vi "Ultrasonic.vi"() -> ()   [LabVIEW 2016, in "ENED1100-UCBA-Sensor-Motor-Testing.lvrbt"]
uses:
  ENED1100-UCBA-Sensor-Motor-Testing.lvrbt
  <vilib>/NXT/Block Support/NXT_InputPort.ctl
  <vilib>/NXT/Subs/LVHSConnector.ctl
  <vilib>/NXT/LegoClasses/BrickReference/BrickReference.lvclass
  <vilib>/NXT/Dual Mode Library/Sensors/EV3_Ultrasonic_CM.vi
  <vilib>/NXT/Dual Mode Library/Sound/PlayF.vi
  <vilib>/NXT/Dual Mode Library/Sound/PlayC.vi
panel:
  out "NXT/EV3 4":T1
  in  "NXT/EV3 3":T1
  in  "Port (Port 3) 2":T2=3 items=["Port 1", "Port 2", "Port 3", "Port 4"]
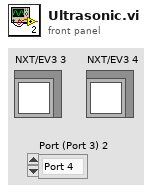
[diagram p1: front panel]
types:
  T1 = typedef "LVHSConnector.ctl" = refnum<class "BrickReference.lvclass">
  T2 = typedef "NXT_InputPort.ctl" = u32
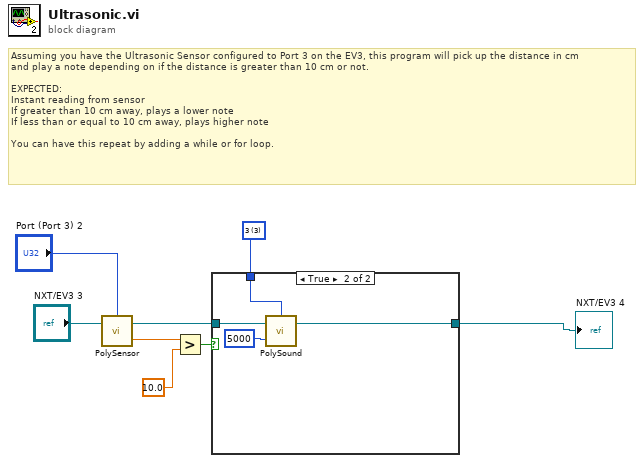
[diagram p0: block diagram]
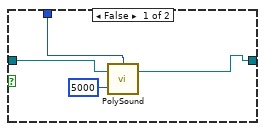
[diagram p2: hidden frame]
diagram:
  w3 = u16 3 items=["3"=3, "4"=4, "5"=5, "6"=6, "7"=7] ("Octave")
  # "Assuming you have the Ultrasonic Sensor configured to Port 3 on the EV3, this program will pick up the distance in cm\nand play a note depending on if the distance is greater than 10 cm or not.\n\nEXPECTED:\nInstant reading from sensor\nIf greater than 10 cm away, plays a lower note\nIf less than or equal to 10 cm away, plays higher note\n\nYou can have this repeat by adding a while or for loop."
  n1 = call-poly <vilib>:"PolySensor.vi"("NXT/EV3"="NXT/EV3 3", "Port (Port 1)"="Port (Port 3) 2") -> ("Centimeters"=w2:sgl, "NXT/EV3"=w5:T1)  [unwired: 1 in]
  n2 = Greater?(x=w2, y=sgl 10.0) -> (0:w6:bool)
  n3 = case shown="True" w6 {
    tunnel: w5 -> [w12 w16]
    tunnel: [w11 w14] -> w4
    tunnel: w3 -> [w10 w13]
    frame False {
      n4 = call-poly <vilib>:"PolySound.vi"("Duration (500 ms)"=u16 5000, "NXT/EV3"=w12, "Octave"=w10) -> ("NXT/EV3"=w11:T1)  [unwired: 1 in]
    }
    frame True {
      n5 = call-poly <vilib>:"PolySound.vi"("Duration (500 ms)"=u16 5000, "NXT/EV3"=w16, "Octave"=w13) -> ("NXT/EV3"=w14:T1)  [unwired: 1 in]
    }
  }
  "NXT/EV3 4" <- w4
